vi "GitNeedsSaveGUI.vi"(4 "Current Save Panel Info":T1, 6 "Diff Input":string, 7 "AuthorRing":refnum<vi>, 8 "error in (no error)":errorcluster, 9 "Save Repo Path":path=path "", 10 "Save Cluster":T2 {"Select Layout" items=["Default"]}, 11 "Git exec":string="git") -> (0 "error out":errorcluster, 1 "Save Repo Path Out":path, 2 "Continue":bool, 3 "Git exec out":string="git", 5 "Saved":bool)   [LabVIEW 2013]
uses:
  TypeDefs/SaveCluster.ctl
  VariableManagerCodes/VariableManager/VariableManager.lvclass
  DeviceVIs/Device/Device.lvclass
  <vilib>/Utility/miscctls.llb/LVStringsAndValuesArrayTypeDef_I32.ctl
panel:
  in  "NoContinueOrSave":bool
  in  "Author":u16(ring) items=["SetList Program <JQIbot@users.noreply.github.com>", "What <even@is.this>"]
  in  "Description":string
  in  "SaveTitle":string caption="Title/Filename"
  in  "ContinueWithoutSaving":bool
  in  "SaveToRepo":bool
  in  "SeeChanges":bool
  # "You are about to run with unsaved changes. \nWould you like to save before continuing?"
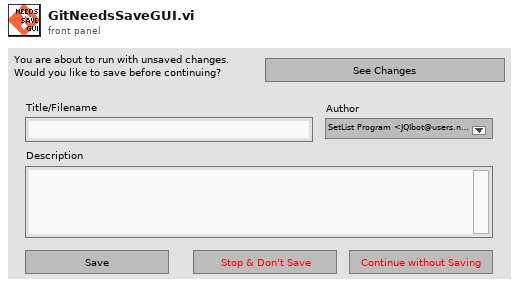
[diagram p1: front panel]
types:
  T1 = cluster{"Title":string, "Description":string, "Author":string}
  T2 = typedef "SaveCluster.ctl" = cluster{"Version":string, "Devices":refnum<class "Device.lvclass">[], "Select Layout":i32, "Layout:Strings And Values []":T3, "User defined functions":string, "VariableManager":refnum<class "VariableManager.lvclass">}
  T3 = typedef "LVStringsAndValuesArrayTypeDef_I32.ctl" = cluster{"String":string, "Value":i32}[]
  T4 = typedef "LVStringsAndValuesArrayTypeDef.ctl" = cluster{"String":string, "Value":ext}[]
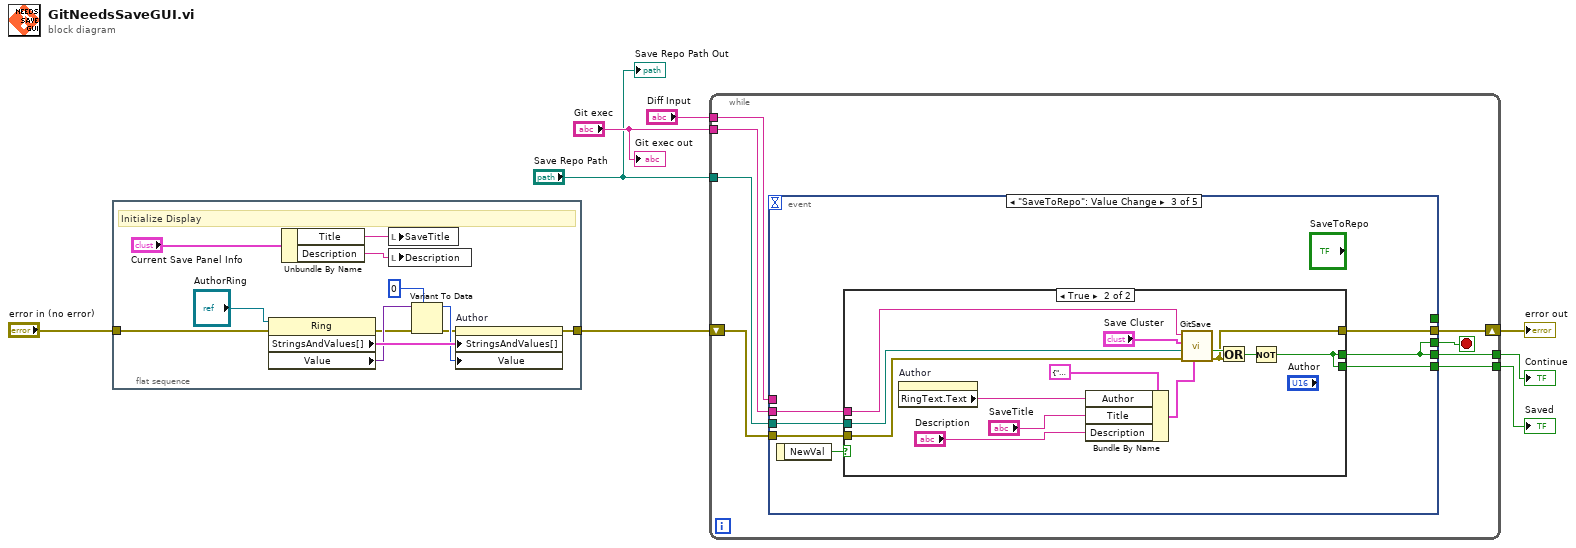
[diagram p0: block diagram]
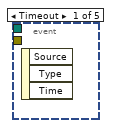
[diagram p2: hidden frame]
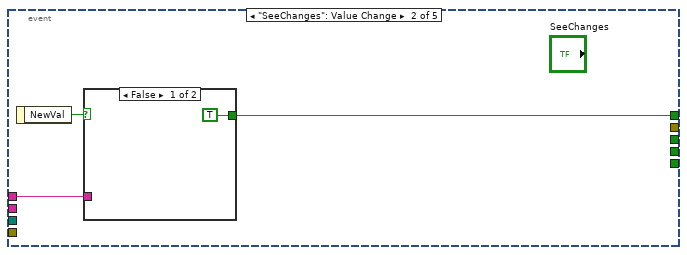
[diagram p3: hidden frame]
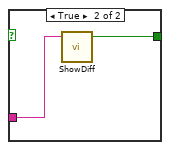
[diagram p4: hidden frame]
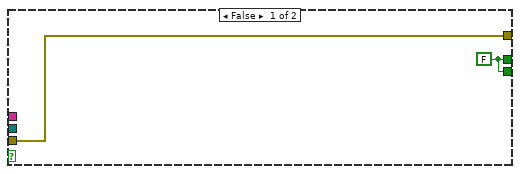
[diagram p5: hidden frame]
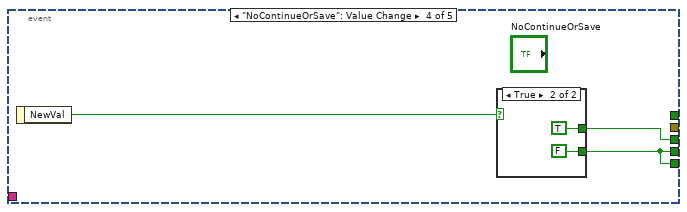
[diagram p6: hidden frame]
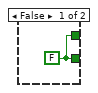
[diagram p7: hidden frame]
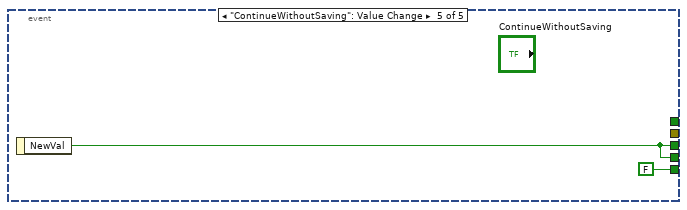
[diagram p8: hidden frame]
diagram:
  n1 = flat-sequence {
    tunnel: "error in (no error)" -> [w19]
    tunnel: [w20] -> w2
    frame #0 {
      # "Initialize Display"
      n2 = property class="Ring"(reference="AuthorRing", error in=w19) -> (error out=w12:errorcluster, "StringsAndValues[]"=w17:T4, "Value"=w16:variant)  [unwired: 1 out]
      n3 = Unbundle By Name("Current Save Panel Info") -> ("Title"=w9:string, "Description"=w10:string)
      n4 = local write "SaveTitle"(w9) -> ()
      n5 = local write "Description"(w10) -> ()
      n6 = Variant To Data(error in=w12, type=u16 0, Variant=w16) -> (data=w15:u16, error out=w13:errorcluster)
      n7 = property on="Author" class="Ring (strict)"(error in=w13, "StringsAndValues[]"=w17, "Value"=w15) -> (error out=w20:errorcluster)  [unwired: 1 in, 1 out]
    }
  }
  n8 = while {
    tunnel: [w28] -> w8
    tunnel: "Diff Input" -> [w26]
    tunnel: "Git exec" -> [w25]
    tunnel: "Save Repo Path" -> [w24]
    shift-right: [w23] -> w4
    shift-left: w2 -> [w22]
    tunnel: [w21] -> w1
    stop <- w27 stop-if-true
    n9 = event shown="[2] \"SaveToRepo\": Value Change" {
      selector: _ -> [_ _ _ _ _]
      dyn-events: _ -> [_ _ _ _ _]
      timeout: _ -> [_ _ _ _ _]
      tunnel: [_ _ w36 w57 w64] -> w28
      tunnel: [_ _ w36 w58 w64] -> w27
      tunnel: w26 -> [_ w30 _ _ _]
      tunnel: w25 -> [_ _ w41 _ _]
      tunnel: w24 -> [_ _ w40 _ _]
      tunnel: [_ _ w39 _ _] -> w23
      tunnel: w22 -> [_ _ w38 _ _]
      tunnel: [_ w29 _ _ _] -> _
      tunnel: [_ _ w35 w57 FALSE] -> w21
      event Timeout {
        n10 = event-data() -> ()  [unwired: 1 in, 3 out]
      }
      event "SeeChanges": Value Change {
        n11 = event-data() -> ("NewVal"=w31:bool)  [unwired: 1 in]
        n12 = case shown="False" w31 {
          tunnel: w30 -> [_ w34]
          tunnel: [TRUE ("UserDone") w33] -> w29
          frame False {
          }
          frame True {
            n13 = call "ShowDiff.vi"("RawDiff"=w34) -> ("UserDone"=w33:bool)  [unwired: 8 in]
          }
        }
      }
      event "SaveToRepo": Value Change {
        n14 = event-data() -> ("NewVal"=w37:bool)  [unwired: 1 in]
        n15 = case shown="True" w37 {
          tunnel: w41 -> [_ w51]
          tunnel: w40 -> [_ w50]
          tunnel: [w43 w46] -> w39
          tunnel: w38 -> [w43 w48]
          tunnel: [w42 w44] -> w36
          tunnel: [w42 w44] -> w35
          frame False {
            w42 = FALSE
          }
          frame True {
            n16 = property on="Author" class="Ring (strict)"() -> ("RingText.Text"=w52:string)  [unwired: 2 in, 2 out]
            n17 = Bundle By Name(cluster=T1 {"Title"="", "Description"="", "Author"=""} ("Commit Meta-Info"), "Author"=w52, "Title"="SaveTitle", "Description"="Description") -> (w56:T1)
            n18 = call "GitSave.vi"("Commit Meta-Info"=w56, "error in (no error)"=w48, "Save Repo Path"=w50, "Save Cluster"="Save Cluster", "Git exec"=w51) -> ("error out"=w46:errorcluster, "User Cancelled"=w47:bool)  [unwired: 3 in, 2 out]
            n19 = Or(x=w47, y=w46) -> (x .or. y?=w45:bool)
            n20 = Not(x=w45) -> (.not. x?=w44:bool)
          }
        }
      }
      event "NoContinueOrSave": Value Change {
        n21 = event-data() -> ("NewVal"=w59:bool)  [unwired: 1 in]
        n22 = case shown="True" w59 {
          tunnel: [w60 TRUE] -> w58
          tunnel: [w60 FALSE] -> w57
          frame False {
            w60 = FALSE
          }
          frame True {
          }
        }
      }
      event "ContinueWithoutSaving": Value Change {
        n23 = event-data() -> ("NewVal"=w64:bool)  [unwired: 1 in]
      }
    }
  }
  "error out" <- w4
  "Continue" <- w8
  "Saved" <- w1
  "Save Repo Path Out" <- "Save Repo Path"
  "Git exec out" <- "Git exec"
